vi "Enqeue message.vi"(8 "error in (no error)":errorcluster, 11 "RxTx in":refnum<class "RxTx.lvclass">) -> (0 "error out":errorcluster, 3 "RxTx out":refnum<class "RxTx.lvclass">)   [LabVIEW 2018, in "RxTx.lvclass"]
doc: "Este VI adiciona um elemento à fila."
uses:
  RxTx.lvclass
  RxTx.lvclass/RxTx.ctl
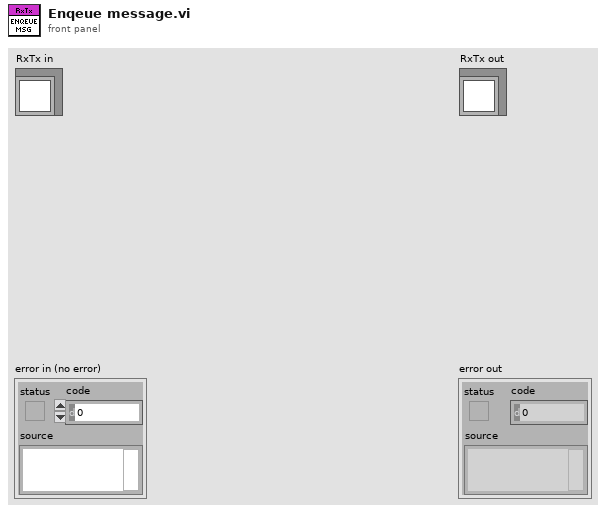
[diagram p1: front panel]
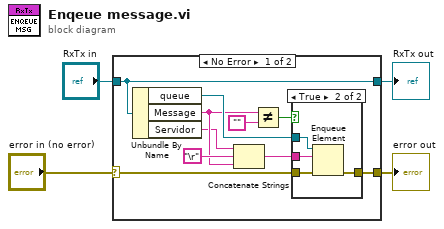
[diagram p0: block diagram]
diagram:
  n1 = case shown="No Error" "error in (no error)" {
    selector: "error in (no error)" -> [w10 w21]
    tunnel: [w13 w21] -> w3
    tunnel: [w9 w20] -> w1
    tunnel: "RxTx in" -> [w9 w20]
    frame No Error {
      n2 = Unbundle By Name(w9) -> ("queue"=w14:refnum<queue>, "Message"=w7:string, "Servidor"=w5:string)
      n3 = Concatenate Strings(w5, "\r", w7) -> (w6:string)
      n4 = Not Equal?(x=w7, y="") -> (x != y?=w12:bool)
      n5 = case shown="True" w12 {
        tunnel: w14 -> [_ w19]
        tunnel: [w15 w18] -> w13
        tunnel: w6 -> [_ w17]
        tunnel: w10 -> [w15 w16]
        frame False {
        }
        frame True {
          n6 = Enqueue Element(queue=w19, element=w17, error in (no error)=w16) -> (error out=w18:errorcluster)  [unwired: 1 in, 2 out]
        }
      }
    }
    frame Error {
    }
  }
  "error out" <- w3
  "RxTx out" <- w1
